vi "Resampling a Waveform (continuous).vi"() -> ()   [LabVIEW 2020]
doc: "This example demonstrates the effect of resampling a waveform in continuous mode, and calculates a power spectrum of the resampled signal."
uses:
  <vilib>/Analysis/4window.llb/windowTd.ctl
  <vilib>/measure/maspectr.llb/FFT Power Spectrum and PSD for 1 Chan.vi
  <vilib>/measure/maresamp.llb/Resample Waveform (continuous).vi
  <vilib>/measure/NI_MABase.lvlib
  <vilib>/measure/NI_MAPro.lvlib
  <vilib>/Analysis/NI_AALPro.lvlib
panel:
  in  "FIR Filter Specifications":T1={"Alias Rejection (dB)"=100.0, "Normalized Bandwidth"=0.4}
  in  "Interpolation Mode":u16(ring)=2 items=["coerce", "linear", "spline", "FIR filter"]
  out "Waveforms":waveform(dbl)[](graph)
  out "Power Spectra (dB)":cluster{"f0":dbl, "df":dbl, "magnitude":dbl[]}[](graph)
  in  "Stop":bool
  # "Overview: Demonstrates the effect of resampling a waveform in continuous mode, and calculates a power spectrum of the resampled signal.\nRequirements: LabVIEW Full Development System\nInstructions:\n1. Run the VI. Observe the differences between the original and resampled waveforms in the graphs.\n2. Click Stop to stop the VI."
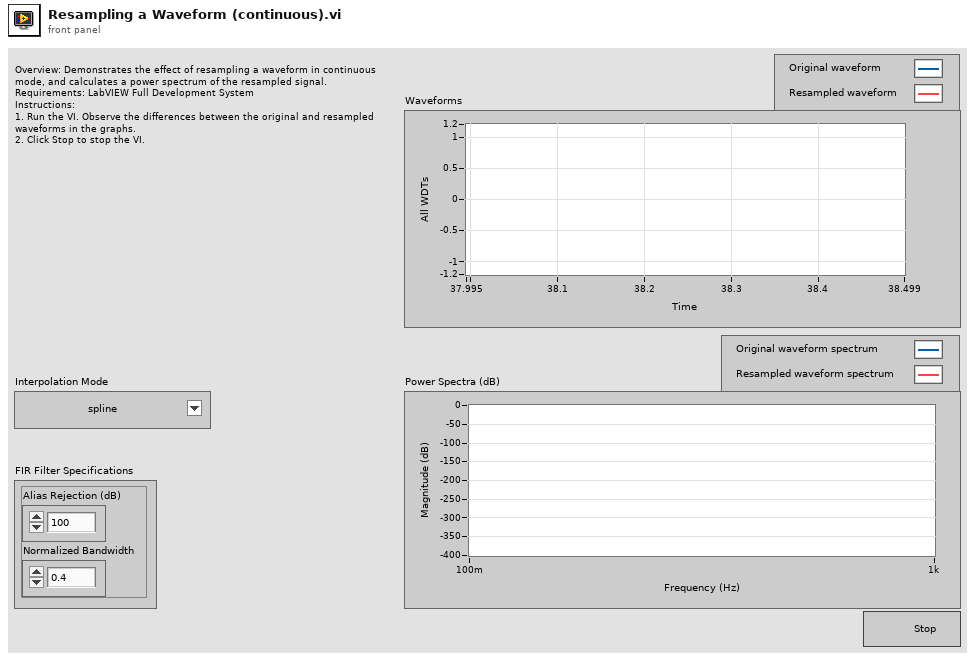
[diagram p1: front panel]
types:
  T1 = cluster{"Alias Rejection (dB)":dbl, "Normalized Bandwidth":dbl}
  T2 = typedef "NI_AALPro.lvlib/windowTd.ctl" = u32
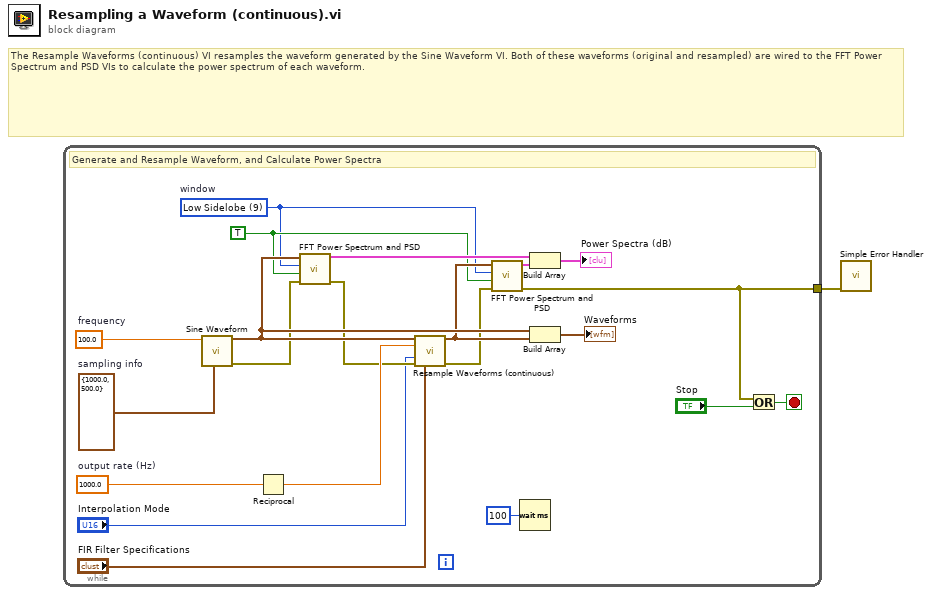
[diagram p0: block diagram]
diagram:
  # "The Resample Waveforms (continuous) VI resamples the waveform generated by the Sine Waveform VI. Both of these waveforms (original and resampled) are wired to the FFT Power Spectrum and PSD VIs to calculate the power spectrum of each waveform."
  n1 = while {
    tunnel: [w4] -> w1
    stop <- w5 stop-if-true
    w16 = 100.0  # frequency
    w15 = cluster{"Fs":dbl, "# s":dbl} {"Fs"=1000.0, "# s"=500.0}  # sampling info
    w14 = 1000.0  # output rate (Hz)
    w7 = T2 9 items=["Rectangle"=0, "Hanning"=1, "Hamming"=2, "Blackman-Harris"=3, "Exact Blackman"=4, "Blackman"=5, "Flat Top"=6, "4 Term B-Harris "=7, "7 Term B-Harris"=8, "Low Sidelobe"=9, "Blackman Nuttall"=11, "Triangle"=30, "Bartlett-Hanning"=31, "Bohman"=32, "Parzen"=33, "Welch"=34, "Kaiser"=60, "Dolph-Chebyshev"=61, "Gaussian"=62]  # window
    w18 = TRUE ("dB On (F)")
    # "Generate and Resample Waveform, and Calculate Power Spectra"
    n2 = call <vilib>:"Sine Waveform.vi"("sampling info"=w15, "frequency"=w16) -> ("error out"=w9:errorcluster, "signal out"=w20:waveform(dbl))  [unwired: 5 in, 3 out]
    n3 = Reciprocal(x=w14) -> (1/x=w13:dbl)
    n4 = call-poly <vilib>:"FFT Power Spectrum and PSD.vi"("error in (no error)"=w9, "dB On (F)"=w18, "window"=w7, "time signal"=w20) -> ("error out"=w8:errorcluster, "Power Spectrum / PSD"=w21:cluster{"f0":dbl, "df":dbl, "magnitude":dbl[]})  [unwired: 4 in, 2 out]
    n5 = call-poly <vilib>:"Resample Waveforms (continuous).vi"("waveform in"=w20, "dt"=w13, "interpolation mode"="Interpolation Mode", "error in (no error)"=w8, "FIR filter specifications"="FIR Filter Specifications") -> ("resampled waveform out"=w19:waveform(dbl), "error out"=w6:errorcluster)  [unwired: 3 in, 6 out]
    n6 = call-poly <vilib>:"FFT Power Spectrum and PSD.vi"("error in (no error)"=w6, "dB On (F)"=w18, "window"=w7, "time signal"=w19) -> ("error out"=w4:errorcluster, "Power Spectrum / PSD"=w17:cluster{"f0":dbl, "df":dbl, "magnitude":dbl[]})  [unwired: 4 in, 2 out]
    n7 = Wait (ms)(milliseconds to wait=u32 100) -> ()  [unwired: 1 out]
    n8 = Build Array(w21, w17) -> (→"Power Spectra (dB)":cluster{"f0":dbl, "df":dbl, "magnitude":dbl[]}[])
    n9 = Build Array(w20, w19) -> (→"Waveforms":waveform(dbl)[])
    n10 = Or(x=w4, y="Stop") -> (x .or. y?=w5:bool)
  }
  n11 = call <vilib>:"Simple Error Handler.vi"("error in (no error)"=w1) -> ()  [unwired: 4 in, 5 out]
